vi "SetProjectConditionalDeactivationValueByKey.vi"(8 "Fehler (Eingang, kein Fehler)":errorcluster, 10 "Tabellen-String":string, 11 "Projekt Referenz":refnum<vi>) -> (0 "Fehler (Ausgang)":errorcluster, 3 "Projekt Referenz":refnum<vi>)   [LabVIEW 2015, in "ConditionalDeactivation.lvlib"]
uses:
  ConditionalDeactivation.lvlib
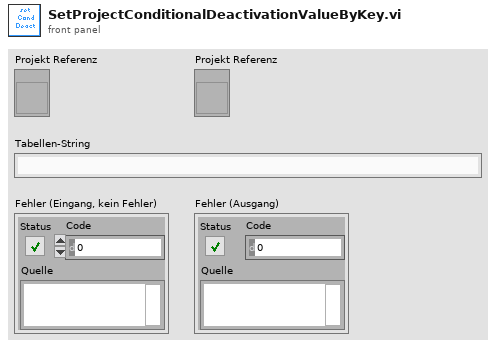
[diagram p1: front panel]
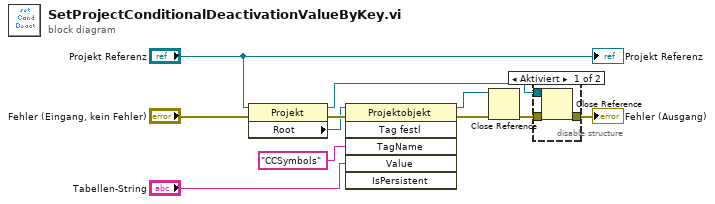
[diagram p0: block diagram]
diagram:
  n1 = property class="Projekt"(reference="Projekt Referenz", error in="Fehler (Eingang, kein Fehler)") -> (reference out=w4:refnum<vi>, error out=w9:errorcluster, "Root"=w8:refnum<vi>)
  n2 = invoke class="Projektobjekt" method="Tag festl"(reference=w8, error in=w9, "TagName"="CCSymbols" ("Tag-Name"), "Value"="Tabellen-String") -> (reference out=w5:refnum<vi>, error out=w2:errorcluster)  [unwired: 2 in, 4 out]
  n3 = Close Reference(reference=w5, error in (no error)=w2) -> (error out=w7:errorcluster)
  n4 = disable-structure shown="Aktiviert" {
    disable-tunnel: w7 -> [w14 w15]
    disable-tunnel: [w13 w15] -> w6
    disable-tunnel: w4 -> [w12 _]
    frame Enabled {
      n5 = Close Reference(reference=w12, error in (no error)=w14) -> (error out=w13:errorcluster)
    }
    frame Disabled {
    }
  }
  "Fehler (Ausgang)" <- w6
  "Projekt Referenz" <- "Projekt Referenz"
